vi "Get Endpoint Configuration.vi"(8 "error in (no error)":errorcluster, 10 "Endpoint":string, 11 "Endpoint Config Section Ref in":T2 format="%.0x") -> (0 "error out":errorcluster, 1 "Endpoint found":bool, 2 "Configuration Type":T1, 3 "Endpoint Config Section Ref out":T2 format="%.0x")   [LabVIEW 2017, in "SLSC Switch Scripting.lvlib"]
uses:
  SLSC Switch Scripting.lvlib
  <vilib>/NI Veristand/Custom Device API/Custom Device Item Ref.ctl
  Endpoint Configuration.ctl
  <vilib>/NI Veristand/Custom Device API/Get Item Property (String).vi
  <vilib>/NI VeriStand/Custom Device API/Custom Device API.lvlib
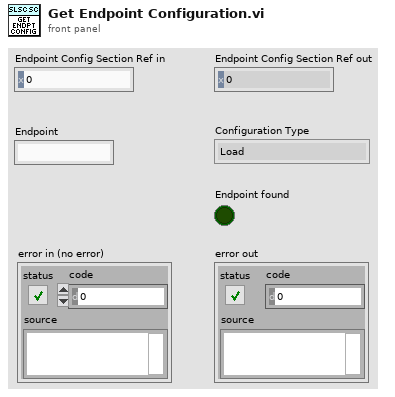
[diagram p1: front panel]
types:
  T1 = typedef "SLSC Switch Scripting.lvlib/Endpoint Configuration.ctl" = enum16{"Load", "Source", "Configuration"}
  T2 = typedef "Custom Device API.lvlib/Custom Device Item Ref.ctl" = u64
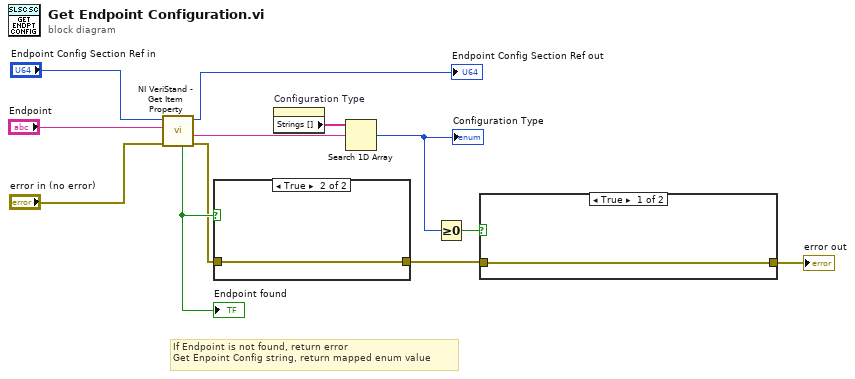
[diagram p0: block diagram]
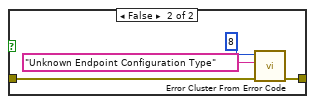
[diagram p2: hidden frame]
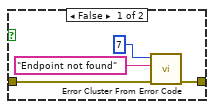
[diagram p3: hidden frame]
diagram:
  # "If Endpoint is not found, return error\nGet Enpoint Config string, return mapped enum value"
  n1 = call-poly <vilib>:"NI VeriStand - Get Item Property.vi"("error in (no error)"="error in (no error)", "Property Name"="Endpoint", "Item Ref in"="Endpoint Config Section Ref in") -> ("error out"=w7:errorcluster, "Value"=w5:string, "Item Ref out"=→"Endpoint Config Section Ref out":T2, "Found?"=w8:bool)  [unwired: 5 in]
  "Endpoint found" <- w8
  n2 = case shown="True" w8 {
    tunnel: w7 -> [w14 w17]
    tunnel: [w13 w17] -> w2
    frame False {
      n3 = call <vilib>:"Error Cluster From Error Code.vi"("error in (no error)"=w14, "error message (\"\")"="Endpoint not found" ("error message (\"\")"), "error code (0)"=7) -> ("error out"=w13:errorcluster)  [unwired: 6 in]
    }
    frame True {
    }
  }
  n4 = property on="Configuration Type" class="Enum (strict)"() -> ("Strings []"=w6:string[])  [unwired: 2 in, 2 out]
  n5 = Search 1D Array(1D array=w6, element=w5) -> (index of element=w3:i32)  [unwired: 1 in]
  "Configuration Type" <- w3
  n6 = Greater Or Equal To 0?(x=w3) -> (x >= 0?=w4:bool)
  n7 = case shown="True" w4 {
    tunnel: [w18 w20] -> w1
    tunnel: w2 -> [w18 w19]
    frame True {
    }
    frame False {
      n8 = call <vilib>:"Error Cluster From Error Code.vi"("error in (no error)"=w19, "error message (\"\")"="Unknown Endpoint Configuration Type" ("error message (\"\")"), "error code (0)"=8) -> ("error out"=w20:errorcluster)  [unwired: 6 in]
    }
  }
  "error out" <- w1
